vi "Sel Biometry Average Attribute.vi"(8 "error in (no error)":errorcluster caption="错误输入（无错误）", 9 "condition":string, 11 "connection reference":T2) -> (0 "error out":errorcluster caption="错误输出", 2 "Biometry Average Attribute":T1[](array[typedef]))   [LabVIEW 2015, in "Database Processing.lvlib"]
doc: "该模板用于创建子VI。"
uses:
  Database Processing.lvlib
  <vilib>/addons/database/Connection.llb/Conn ObjectReference.ctl
  Support/Table/Biometry Average Attribute.ctl
  <vilib>/addons/database/_DB Variant To Data/Database Variant To Data.xnode
  <vilib>/addons/database/NI_Database_API.lvlib
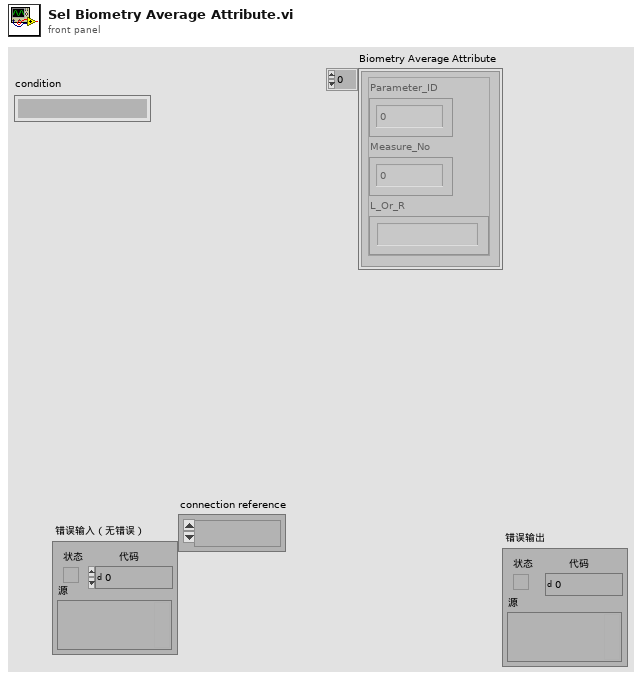
[diagram p1: front panel]
types:
  T1 = typedef "Database Processing.lvlib/Biometry Average Attribute.ctl" = cluster{"Parameter_ID":i64, "Measure_No":i64, "L_Or_R":string}
  T2 = typedef "NI_Database_API.lvlib/Conn ObjectReference.ctl" = refnum<k1>
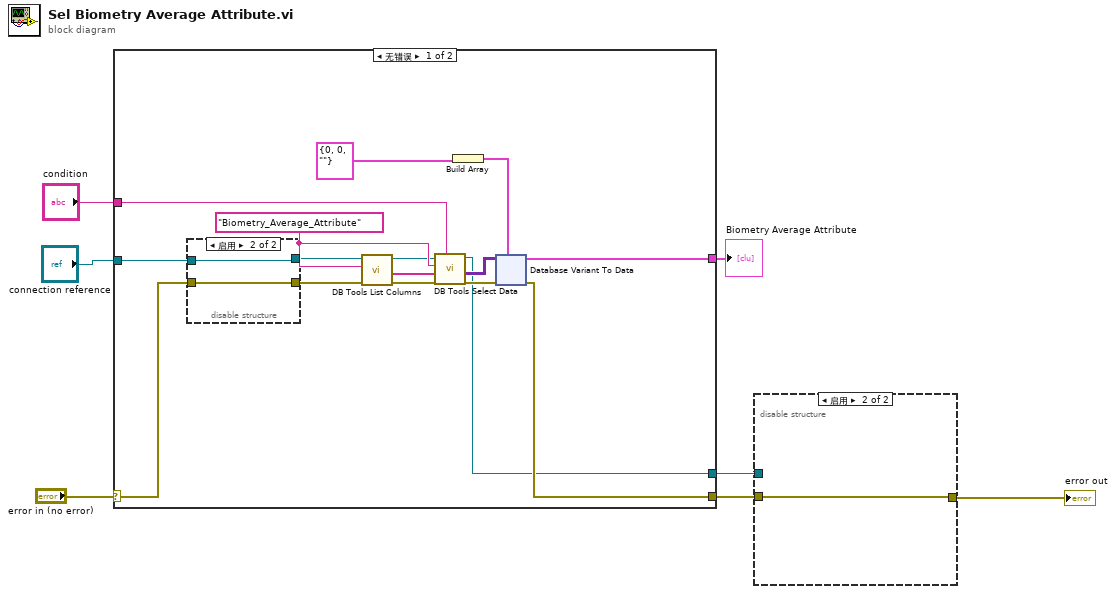
[diagram p0: block diagram]
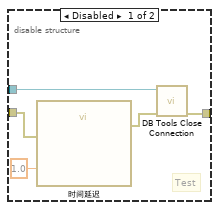
[diagram p2: hidden frame]
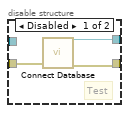
[diagram p3: hidden frame]
diagram:
  n1 = case shown="无错误" "error in (no error)" {
    selector: "error in (no error)" -> [w11 w133]
    tunnel: [w20 w133] -> w3
    tunnel: "connection reference" -> [w13 w132]
    tunnel: [w16 _] -> w1
    tunnel: "condition" -> [w15 _]
    tunnel: [w9 w132] -> w4
    frame No Error {
      w17 = "Biometry_Average_Attribute" ("table")
      n2 = disable-structure shown="启用" {
        disable-tunnel: [w26 w28] -> w14
        disable-tunnel: w13 -> [_ w28]
        disable-tunnel: w11 -> [w25 w27]
        disable-tunnel: [w24 w27] -> w12
        frame Disabled {
          # "Test"
          n3 = call "Connect Database.vi"("error in (no error)"=w25) -> ("error out"=w24:errorcluster, "connection reference"=w26:T2)  [unwired: 9 in]
        }
        frame Enabled {
        }
      }
      n4 = call <vilib>:"DB Tools List Columns.vi"("error in (no error)"=w12, "table"=w17, "connection reference"=w14) -> ("error out"=w19:errorcluster, "columns"=w18:string[], "connection reference out"=w10:T2)  [unwired: 1 in, 1 out]
      n5 = call <vilib>:"DB Tools Select Data.vi"("condition"=w15, "error in (no error)"=w19, "columns"=w18, "table"=w17, "connection reference"=w10) -> ("error out"=w23:errorcluster, "data"=w22:variant[][], "connection reference out"=w9:T2)  [unwired: 1 in]
      n6 = Build Array(T1 {"Parameter_ID"=0, "Measure_No"=0, "L_Or_R"=""} ("Biometry Average Attribute")) -> (w21:T1[])
      n7 = xnode "Database Variant To Data"("database variant"=w22, "error in (no error)"=w23, "type"=w21) -> ("data"=w16:T1[], "error out"=w20:errorcluster)
    }
    frame Error {
    }
  }
  "Biometry Average Attribute" <- w1
  n8 = disable-structure shown="启用" {
    disable-tunnel: w3 -> [w136 w139]
    disable-tunnel: [w138 w139] -> w2
    disable-tunnel: w4 -> [w137 _]
    frame Disabled {
      # "Test"
      n9 = call "时间延迟"("error in (no error)"=w136, "Delay Time (s)"=1.0) -> ("error out"=w135:errorcluster)  [unwired: 9 in]
      n10 = call <vilib>:"DB Tools Close Connection.vi"("error in (no error)"=w135, "connection reference"=w137) -> ("error out"=w138:errorcluster)  [unwired: 5 in]
    }
    frame Enabled {
    }
  }
  "error out" <- w2
